vi "ACTION.vi"() -> ()   [LabVIEW 2017]
panel:
  out "ACTION":string
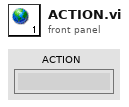
[diagram p1: front panel]
diagram:
